vi "i q sum 2 spc.vi"(9 "input valid":bool=TRUE, 10 "IQ in 2":T1[](array[typedef])=[{"I"=0.0, "Q"=0.0, "overflow"=FALSE}, {"I"=0.0, "Q"=0.0, "overflow"=FALSE}], 11 "IQ in":T1[](array[typedef])=[{"I"=0.0, "Q"=0.0, "overflow"=FALSE}, {"I"=0.0, "Q"=0.0, "overflow"=FALSE}]) -> (2 "output valid":bool, 3 "IQ out":T1[](array[typedef]))   [LabVIEW 2021]
doc: "sum 2 IQ datas (I+I =>I ; Q+Q =>Q ; overflow or overflow or +overflow => overflow"
uses:
  <instrlib>/_niInstr/DSP/v1/Shared/Public/IQ Data.ctl
  <instrlib>/_niInstr/DSP/v1/Shared/niInstr DSP v1 Shared.lvlib
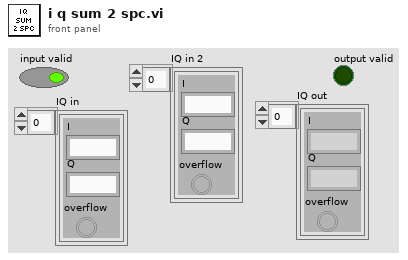
[diagram p1: front panel]
types:
  T1 = typedef "niInstr DSP v1 Shared.lvlib/IQ Data.ctl" = cluster{"I":fxp<+/-,18,1>, "Q":fxp<+/-,18,1>, "overflow":bool}
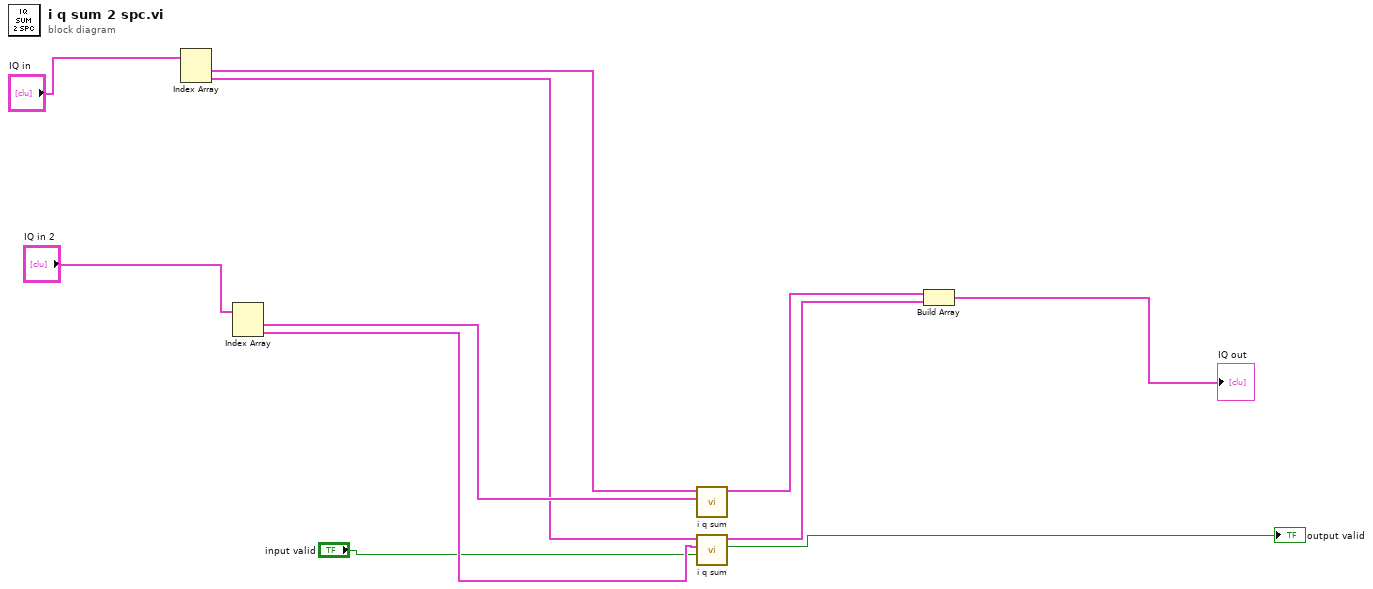
[diagram p0: block diagram]
diagram:
  n1 = Index Array(array="IQ in") -> (element #1=w1:T1, element #2=w2:T1)  [unwired: 2 in]
  n2 = Index Array(array="IQ in 2") -> (element #1=w9:T1, element #2=w8:T1)  [unwired: 2 in]
  n3 = call "i q sum.vi"(10:"data in"=w9, 11:"data in"=w1) -> ("output cluster"=w7:T1)  [unwired: 8 in, 1 out]
  n4 = call "i q sum.vi"("input valid"="input valid", 10:"data in"=w8, 11:"data in"=w2) -> ("output valid"=→"output valid":bool, "output cluster"=w6:T1)  [unwired: 7 in]
  n5 = Build Array(w7, w6) -> (→"IQ out":T1[])
